vi "IMAQDevice.publish_data.vi"(0 "i ref in":refnum<vi>, 5 "error in (no error)":errorcluster) -> (14 "i ref out":refnum<vi>, 19 "error out":errorcluster)   [LabVIEW 2014, in "IMAQDevice.lvlib"]
doc: "This VI publishes data of recently aqcuired images via DIM.\n\nLicense Agreement for this software:\n\nCopyright (C)\nGesellschaft für Schwerionenforschung, GSI\nPlanckstr. 1\n64291 Darmstadt\nGermany\n\nContact: D.Beck@gsi.de \n\nThis program is free software; you can redistribute it and/or modify it under the terms of the \nGNU General Public License as published by the Free Software Foundation; either version 2 of \nthe license, or (at your option) any later version.\n\nThis program is distributed in the hope that it will be useful, but WITHOUT ANY WARRANTY; \nwithout even the implied warranty of MERCHANTABILITY or FITNESS FOR A PARTICULAR PURPOSE. See the GNU General License for more details (http://www.gnu.org).\n\nGesellschaft für Schwerionenforschung, GSI\nPlanckstr. 1, 64291 Darmstadt, Germany\nFor all questions and ideas contact: M.Richter@gsi.de, H.Brand@gsi.de or D.Beck@gsi.de.\nLast update: 16-JUN-2004"
uses:
  IMAQDevice.lvlib
  CSlibraries-extern/DimLVEvent/LVDimInterface/LVDimInterface.lvlib
  CSlibraries/UtilityLib/UtilityLib.lvlib
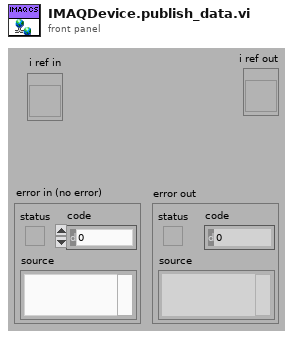
[diagram p1: front panel]
types:
  T1 = typedef "IMAQDevice.lvlib/IMAQDevice.i attribute.ctl" = cluster{"HGF_IMAQ.lvlib:HGF_IMAQDevice.lvclass":refnum<class "HGF_IMAQDevice.lvclass">, "Image":T2, "TimeStampID":i32, "Image IDs":i32[], "NumberOfImagesID":i32, "JPEG?":bool, "JPEGID":i32, "JPEG_ImageID":i32, "TriggerModeID":i32, "OffsetFromLeft":i32, "OffsetFromTop":i32, "HorizontalPixelPerMm":dbl, "VerticalPixelPerMm":dbl, "Grid":cluster{"1":cluster{i32, i32}, "2":cluster{i32, i32}, "3":cluster{i32, i32}, "4":cluster{i32, i32}}, "GridR":cluster{"1":cluster{dbl, dbl}, "2":cluster{dbl, dbl}, "3":cluster{dbl, dbl}, "4":cluster{dbl, dbl}}, "CameraTypeID":i32, "CameraInfos":cluster{"Camera Name-Array":string[], "own Camera Type":string}, "TakeMeasurement?":bool, "TriggerArmedID":i32, "Mirroring":i16, "Rotation":dbl}
  T2 = typedef "IMAQ Image.ctl" = refnum<image>
  T3 = typedef "LVDateTimeRec.ctl" = cluster{"fractional second":dbl, "second":i32, "minute":i32, "hour":i32, "day of month":i32, "month":i32, "year":i32, "day of week":i32, "day of year":i32, "DST":i32}
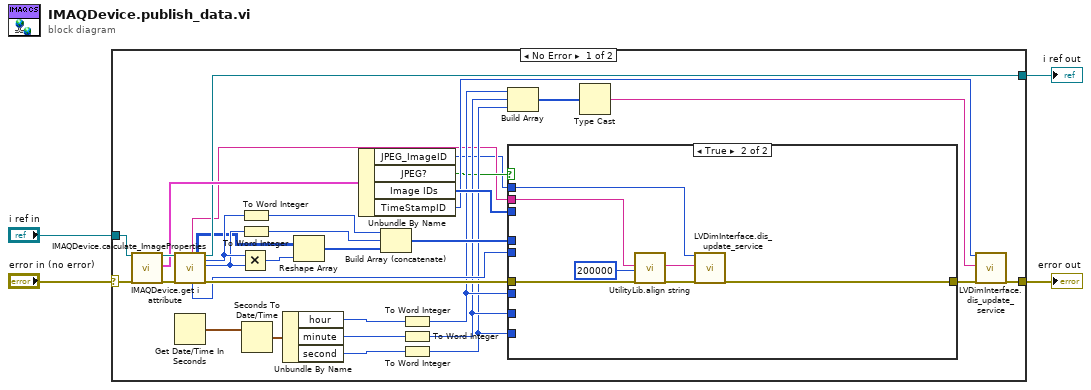
[diagram p0: block diagram]
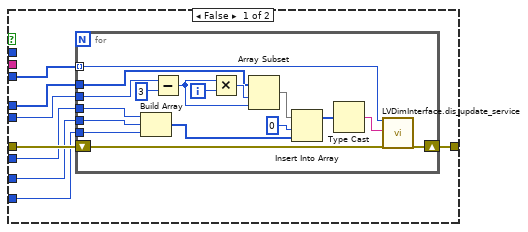
[diagram p2: hidden frame]
diagram:
  n1 = case shown="No Error" "error in (no error)" {
    selector: "error in (no error)" -> [w36 w71]
    tunnel: "i ref in" -> [w37 w70]
    tunnel: [w14 w71] -> w2
    tunnel: [w23 w70] -> w1
    frame No Error {
      n2 = call "IMAQDevice.get i attribute.vi"("i ref in"=w37, "error in (no error)"=w36) -> ("i ref out"=w35:refnum<vi>, "i attribute"=w25:T1, "error out"=w34:errorcluster)  [unwired: 15 in]
      n3 = call "IMAQDevice.calculate_ImageProperties.vi"("i ref in"=w35, "error in (no error)"=w34) -> ("JPEG Image"=w6:string, "length per DIM service / 16 Bit"=w18:i32, "Image Pixels (U8)"=w17:u8[][], "i ref out"=w23:refnum<vi>, "Image hight"=w21:i32, "Image width"=w20:i32, "error out"=w24:errorcluster)  [unwired: 8 in, 3 out]
      n4 = Get Date/Time In Seconds() -> (seconds since 1Jan1904=w29:timestamp)
      n5 = Multiply(x=w21, y=w20) -> (x*y=w19:i32)
      n6 = To Word Integer(number=w21) -> (16bit integer=w28:i16)
      n7 = To Word Integer(number=w20) -> (16bit integer=w27:i16)
      n8 = Seconds To Date/Time(time stamp (now)=w29) -> (date time rec=w30:T3)  [unwired: 1 in]
      n9 = Unbundle By Name(w30) -> ("hour"=w31:i32, "minute"=w32:i32, "second"=w33:i32)
      n10 = Reshape Array(w17, w19) -> (w22:u8[])
      n11 = Unbundle By Name(w25) -> ("JPEG_ImageID"=w5:i32, "JPEG?"=w7:bool, "Image IDs"=w16:i32[], "TimeStampID"=w13:i32)
      n12 = Build Array (concatenate)(w28, w27, w22) -> (w26:i16[])
      n13 = To Word Integer(number=w31) -> (16bit integer=w12:i16)
      n14 = To Word Integer(number=w32) -> (16bit integer=w11:i16)
      n15 = To Word Integer(number=w33) -> (16bit integer=w10:i16)
      n16 = Build Array(w12, w11, w10) -> (w9:i16[])
      n17 = case shown="True" w7 {
        tunnel: w26 -> [w45 _]
        tunnel: w24 -> [w44 w67]
        tunnel: w18 -> [w43 _]
        tunnel: w16 -> [w42 _]
        tunnel: [w41 w69] -> w15
        tunnel: w12 -> [w40 _]
        tunnel: w11 -> [w39 _]
        tunnel: w10 -> [w38 _]
        tunnel: w6 -> [_ w66]
        tunnel: w5 -> [_ w68]
        frame False {
          n18 = for {
            tunnel: w42 -> [w51] mode=indexing
            shift-right: [w49] -> w41
            shift-left: w44 -> [w50]
            tunnel: w43 -> [w61]
            tunnel: w45 -> [w59]
            tunnel: w40 -> [w55]
            tunnel: w39 -> [w52]
            tunnel: w38 -> [w54]
            i -> [w53]
            n19 = Build Array(w55, w52, w54) -> (w56:i16[])
            n20 = Subtract(x=w61, y=3) -> (x-y=w58:i32)
            n21 = Multiply(x=w58, y=w53) -> (x*y=w62:i32)
            n22 = Array Subset(array=w59, index=w62, length=w58) -> (w47:i16[])
            n23 = Insert Into Array(array=w47, index=0, new element=w56) -> (w46:i16[])
            n24 = Type Cast(x=w46) -> (*(type *) &x=w48:string)  [unwired: 1 in]
            n25 = call "LVDimInterface.dis_update_service.vi"("my_serviceID"=w51, "data"=w48, "error in (no error)"=w50) -> ("error out"=w49:errorcluster)  [unwired: 14 in, 2 out]
          }
        }
        frame True {
          n26 = call "UtilityLib.align string.vi"("stringIn"=w66, "stringLength (80)"=200000, "error in (no error)"=w67) -> ("stringOut"=w64:string, "error out"=w65:errorcluster)  [unwired: 15 in]
          n27 = call "LVDimInterface.dis_update_service.vi"("my_serviceID"=w68, "data"=w64, "error in (no error)"=w65) -> ("error out"=w69:errorcluster)  [unwired: 14 in, 2 out]
        }
      }
      n28 = Type Cast(x=w9) -> (*(type *) &x=w8:string)  [unwired: 1 in]
      n29 = call "LVDimInterface.dis_update_service.vi"("my_serviceID"=w13, "data"=w8, "error in (no error)"=w15) -> ("error out"=w14:errorcluster)  [unwired: 14 in, 2 out]
    }
    frame Error {
    }
  }
  "i ref out" <- w1
  "error out" <- w2
